vi "第一个项目.vi"() -> ()   [LabVIEW 2017]
panel:
  in  "停止":bool
  out "波形图表":dbl(graph)
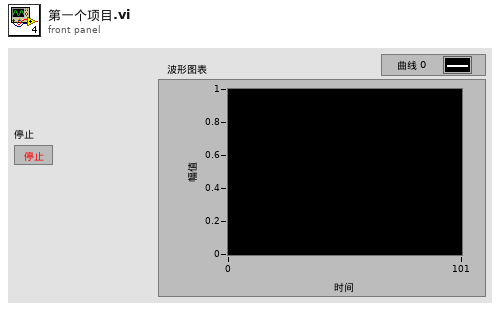
[diagram p1: front panel]
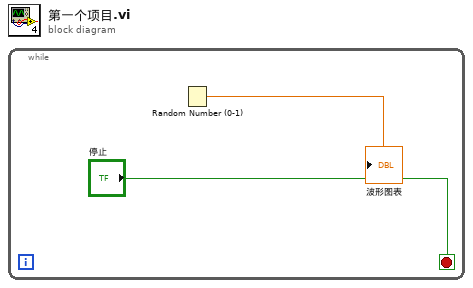
[diagram p0: block diagram]
diagram:
  n1 = while {
    stop <- "停止" stop-if-true
    n2 = Random Number (0-1)() -> (number: 0 to 1=→"波形图表":dbl)
  }
